vi "Convert_Position.vi"(2 "16진수 문자열":string) -> (0 "숫자형":i32)   [LabVIEW 2010]
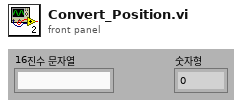
[diagram p1: front panel]
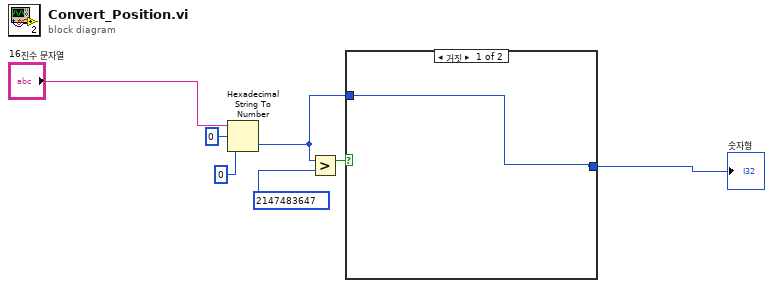
[diagram p0: block diagram]
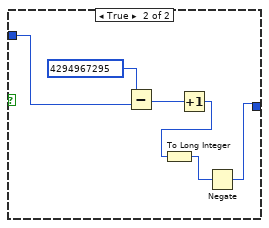
[diagram p2: hidden frame]
diagram:
  n1 = Hexadecimal String To Number(string="16진수 문자열", offset=0 ("오프셋"), default (0uL)=0 ("기본(0 U32)")) -> (number=w2:i32)  [unwired: 1 out]
  n2 = Greater?(x=w2, y=2147483647) -> (0:w3:bool)
  n3 = case shown="거짓" w3 {
    tunnel: w2 -> [w8 w13]
    tunnel: [w8 w9] -> w1
    frame False {
    }
    frame True {
      n4 = Subtract(x=u32 4294967295, y=w13) -> (x-y=w12:u32)
      n5 = Increment(x=w12) -> (x+1=w10:u32)
      n6 = To Long Integer(number=w10) -> (32bit integer=w11:i32)
      n7 = Negate(x=w11) -> (-x=w9:i32)
    }
  }
  "숫자형" <- w1
